vi "getXY.vi"(0 "reference":refnum<class "Direction.lvclass">, 5 "error in (no error)":errorcluster) -> (14 "reference out":refnum<class "Direction.lvclass">, 15 "x":dbl format="%.2f", 16 "y":dbl format="%.2f", 19 "error out":errorcluster)   [LabVIEW 2020, in "Direction.lvclass"]
doc: "public double getX()\nand\npublic double getY()"
uses:
  <resource>/Framework/Providers/Open_GDS/UML/Direction_class/Direction.lvclass
  <resource>/Framework/Providers/Open_GDS/UML/Direction_class/Direction.lvclass/Direction.ctl
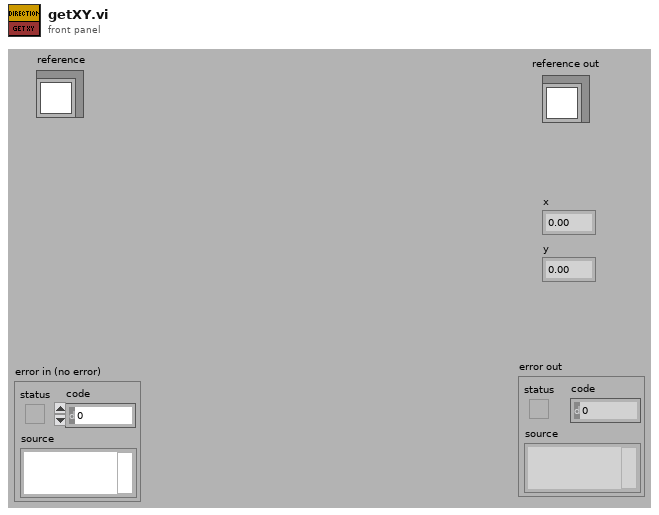
[diagram p1: front panel]
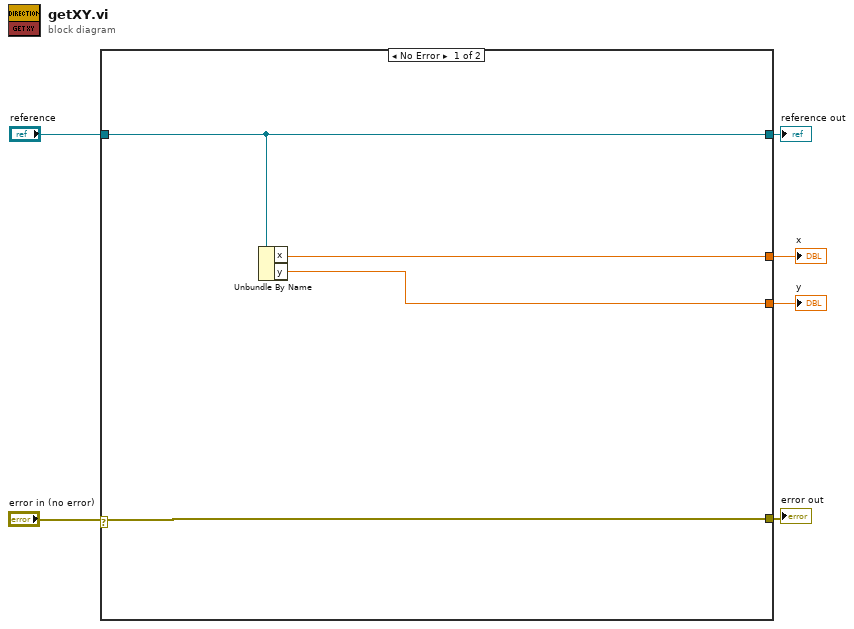
[diagram p0: block diagram]
diagram:
  n1 = case shown="No Error" "error in (no error)" {
    selector: "error in (no error)" -> [w8 w11]
    tunnel: "reference" -> [w7 w12]
    tunnel: [w8 w11] -> w5
    tunnel: [w7 w12] -> w4
    tunnel: [w10 _] -> w2
    tunnel: [w9 _] -> w1
    frame No Error {
      n2 = Unbundle By Name(w7) -> ("x"=w10:dbl, "y"=w9:dbl)
    }
    frame Error {
    }
  }
  "reference out" <- w4
  "error out" <- w5
  "x" <- w2
  "y" <- w1
